vi "DDS_updateManualSettings.vi"() -> ()   [LabVIEW 2012, in "DDS9954_v2013.lvlib"]
uses:
  DDS9954_v2013.lvlib
panel:
  out "FT_Status":u32[](array[numeric])
  out "Bytes Written":u32[](array[numeric])
  in  "Program All DDS?":bool
  in  "Manual Settings Array":T1(array[cluster])=[{"Manual Frequency (MHz)"=110.0, "Manual Amplitude (0-1)"=0.38, "Max Locked Amplitude (0-1)"=0.38, "PD Set-Point (V)"=1.1, "Photodiode Offset (V)"=0.0, "P Gain (-2^8 to 2^8)"=0, "I Gain (-2^8 to 2^8)"=255, "Device Description"="Ultracool FPGA 04", "Gain Divisor (shift << by xBits))"=10, "Nickname"="Dipole 1"}, {"Manual Frequency (MHz)"=75.2, "Manual Amplitude (0-1)"=0.55, "Max Locked Amplitude (0-1)"=0.55, "PD Set-Point (V)"=1.2, "Photodiode Offset (V)"=0.0, "P Gain (-2^8 to 2^8)"=0, "I Gain (-2^8 to 2^8)"=255, "Device Description"="Ultracool FPGA 08", "Gain Divisor (shift << by xBits))"=10, "Nickname"="Dipole 2"}, {"Manual Frequency (MHz)"=92.97, "Manual Amplitude (0-1)"=0.34, "Max Locked Amplitude (0-1)"=0.34, "PD Set-Point (V)"=2.06, "Photodiode Offset (V)"=0.0, "P Gain (-2^8 to 2^8)"=0, "I Gain (-2^8 to 2^8)"=250, "Device Description"="Ultracool FPGA 05", "Gain Divisor (shift << by xBits))"=10, "Nickname"="x-y lattice"}, {"Manual Frequency (MHz)"=91.7, "Manual Amplitude (0-1)"=0.25, "Max Locked Amplitude (0-1)"=0.25, "PD Set-Point (V)"=0.46, "Photodiode Offset (V)"=0.0, "P Gain (-2^8 to 2^8)"=0, "I Gain (-2^8 to 2^8)"=250, "Device Description"="Ultracool FPGA 06", "Gain Divisor (shift << by xBits))"=10, "Nickname"="vertical lattice"}, {"Manual Frequency (MHz)"=0.0, "Manual Amplitude (0-1)"=0.0, "Max Locked Amplitude (0-1)"=0.0, "PD Set-Point (V)"=0.0, "Photodiode Offset (V)"=0.0, "P Gain (-2^8 to 2^8)"=0, "I Gain (-2^8 to 2^8)"=0, "Device Description"="Ultracool FPGA 03", "Gain Divisor (shift << by xBits))"=10, "Nickname"="RF"}, {"Manual Frequency (MHz)"=0.0, "Manual Amplitude (0-1)"=0.0, "Max Locked Amplitude (0-1)"=0.0, "PD Set-Point (V)"=0.0, "Photodiode Offset (V)"=0.0, "P Gain (-2^8 to 2^8)"=0, "I Gain (-2^8 to 2^8)"=0, "Device Description"="Ultracool FPGA 07", "Gain Divisor (shift << by xBits))"=10, "Nickname"="uW Primary"}, {"Manual Frequency (MHz)"=110.0, "Manual Amplitude (0-1)"=0.38, "Max Locked Amplitude (0-1)"=0.38, "PD Set-Point (V)"=1.1, "Photodiode Offset (V)"=0.0, "P Gain (-2^8 to 2^8)"=0, "I Gain (-2^8 to 2^8)"=255, "Device Description"="FPGA 13 uW2", "Gain Divisor (shift << by xBits))"=10, "Nickname"="uW Aux"}, {"Manual Frequency (MHz)"=80.0, "Manual Amplitude (0-1)"=0.0, "Max Locked Amplitude (0-1)"=0.0, "PD Set-Point (V)"=0.0, "Photodiode Offset (V)"=0.0, "P Gain (-2^8 to 2^8)"=0, "I Gain (-2^8 to 2^8)"=0, "Device Description"="Ultracool FPGA", "Gain Divisor (shift << by xBits))"=10, "Nickname"="Running Lattice 1"}, {"Manual Frequency (MHz)"=120.0, "Manual Amplitude (0-1)"=0.33, "Max Locked Amplitude (0-1)"=0.33, "PD Set-Point (V)"=0.0, "Photodiode Offset (V)"=0.0, "P Gain (-2^8 to 2^8)"=0, "I Gain (-2^8 to 2^8)"=0, "Device Description"="FPGA 10 780 Lattice 2", "Gain Divisor (shift << by xBits))"=10, "Nickname"="Running Lattice 2"}, {"Manual Frequency (MHz)"=0.0, "Manual Amplitude (0-1)"=0.0, "Max Locked Amplitude (0-1)"=0.0, "PD Set-Point (V)"=0.0, "Photodiode Offset (V)"=0.0, "P Gain (-2^8 to 2^8)"=0, "I Gain (-2^8 to 2^8)"=0, "Device Description"="FPGA 09", "Gain Divisor (shift << by xBits))"=10, "Nickname"="Bonus FPGA 1"}] {"Manual Frequency (MHz)" min=0.0 max=200.0; "Manual Amplitude (0-1)" min=0.0 max=1.0; "Max Locked Amplitude (0-1)" min=0.0 max=1.0; "PD Set-Point (V)" min=0.0 max=3.3; "Photodiode Offset (V)" min=0.0 max=3.3; "P Gain (-2^8 to 2^8)" min=0 max=255 step=1; "I Gain (-2^8 to 2^8)" min=0 max=255 step=1; "Gain Divisor (shift << by xBits))" max=10 step=1}
  in  "Use DDS display equivalent?":bool
  out "error out":errorcluster
  out "Characters to FPGA":string="L;004\r\nL102200242\r\nL2000034\r\nL01\r\nL411<71<720::::::;0::::::;071<71<7\r\nL615555555155555550>38>38>0>38>38>\r\nL31000100010001000\r\nL50000000000000000\r\nL70200000001010000000102000000010200000001\r\nL80200000001010000000102000000010200000001\r\nL:0;>;<2000;>;<2000;>;<2000;>;<200\r\nL91010\r\n"
  # "Program will reprogram first displayed FPGA device in the array\nAlternatively, program can reprogram ALL FPGA devices by clicking the option"
  # "Nicknames:\nUltracool FPGA 03 = RF\nUltracool FPGA 04 = Dipole 1\nUltracool FPGA 07 = uW 1\nUltracool FPGA 08 = Dipole 2\nFPGA 13 uW2 = uW 2"
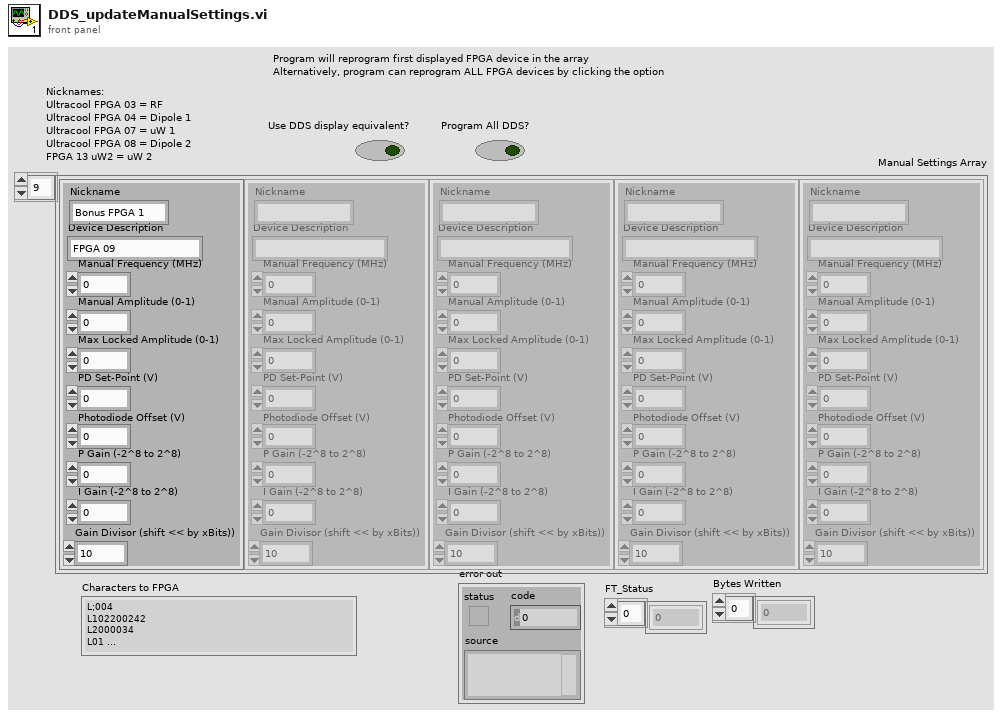
[diagram p1: front panel]
types:
  T1 = cluster{"Manual Frequency (MHz)":dbl, "Manual Amplitude (0-1)":dbl, "Max Locked Amplitude (0-1)":dbl, "PD Set-Point (V)":dbl, "Photodiode Offset (V)":dbl, "P Gain (-2^8 to 2^8)":i16, "I Gain (-2^8 to 2^8)":i16, "Device Description":string, "Gain Divisor (shift << by xBits))":u8, "Nickname":string}[]
  T2 = cluster{"Manual Frequency (MHz)":dbl, "Manual Amplitude (0-1)":dbl, "Max Locked Amplitude (0-1)":dbl, "PD Set-Point (V)":dbl, "Photodiode Offset (V)":dbl, "P Gain (-2^8 to 2^8)":i16, "I Gain (-2^8 to 2^8)":i16, "Device Description":string, "Gain Divisor (shift << by xBits))":u8, "Nickname":string}
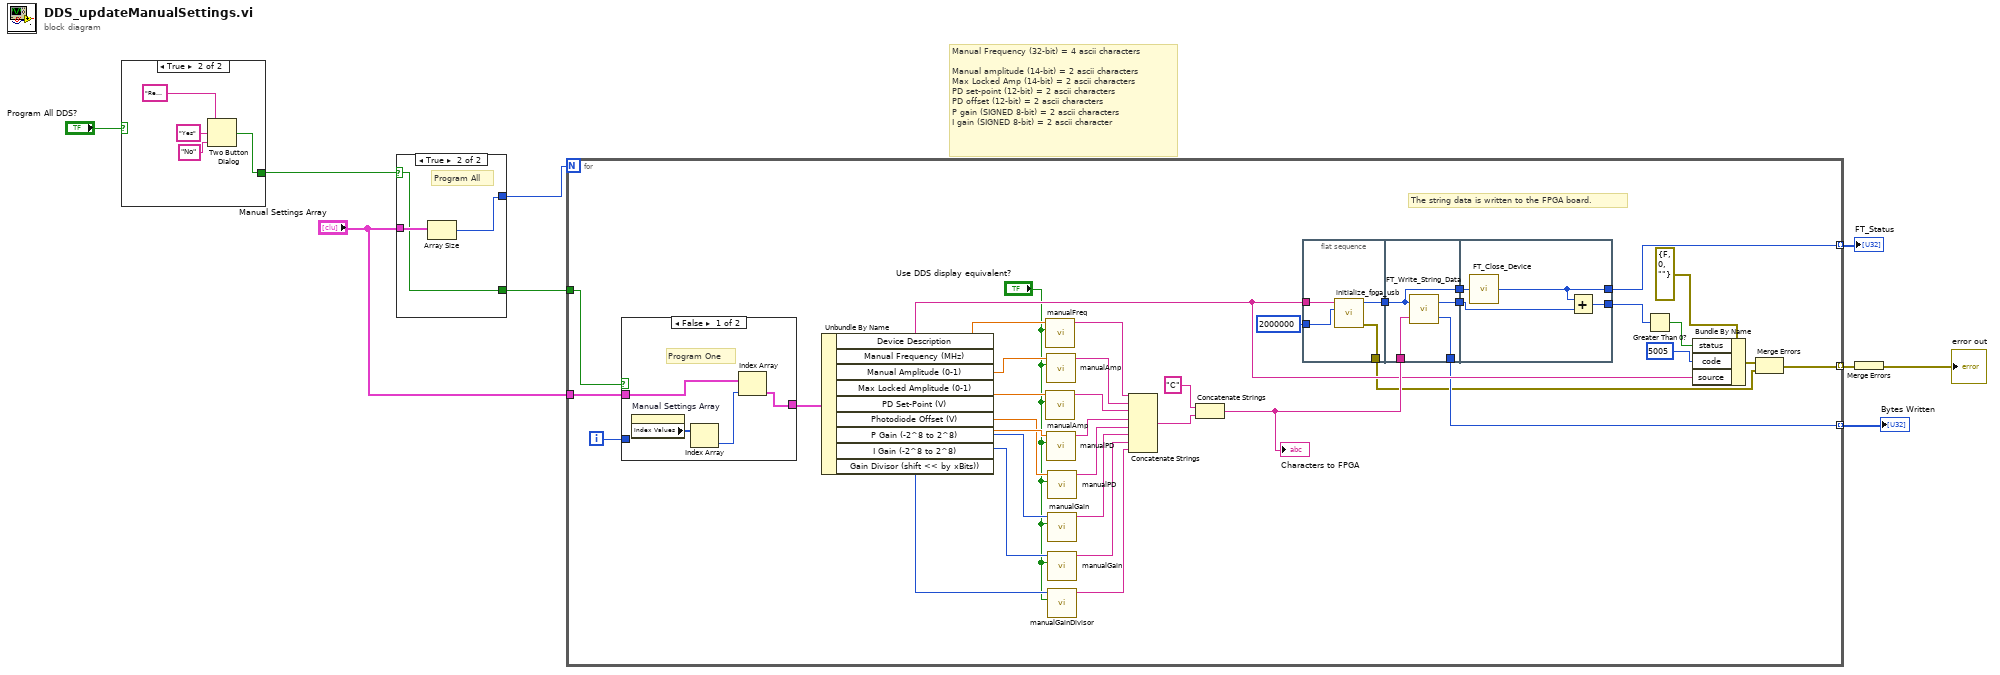
[diagram p0: block diagram]
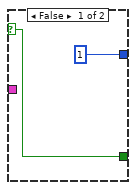
[diagram p3: hidden frame]
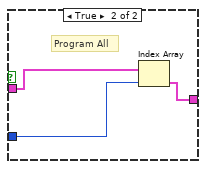
[diagram p4: hidden frame]
diagram:
  # "Manual Frequency (32-bit) = 4 ascii characters\n\nManual amplitude (14-bit) = 2 ascii characters\nMax Locked Amp (14-bit) = 2 ascii characters\nPD set-point (12-bit) = 2 ascii characters\nPD offset (12-bit) = 2 ascii characters\nP gain (SIGNED 8-bit) = 2 ascii characters\nI gain (SIGNED 8-bit) = 2 ascii character"
  n1 = case shown="True" "Program All DDS?" {
    selector: "Program All DDS?" -> [w10 _]
    tunnel: [w10 w14] -> w5
    frame False {
    }
    frame True {
      n2 = Two Button Dialog(message="Really reprogram ALL FPGAs in the array?", 1:"No" ("F button name (\"Cancel\")"), 2:"Yes" ("T button name (\"OK\")")) -> (T button?=w14:bool)
    }
  }
  n3 = case shown="True" w5 {
    selector: w5 -> [w15 w17]
    tunnel: "Manual Settings Array" -> [_ w19]
    tunnel: [1 w18] -> w9
    tunnel: [w15 w17] -> w8
    frame False {
    }
    frame True {
      # "Program All"
      n4 = Array Size(array=w19) -> (size(s)=w18:i32)
    }
  }
  n5 = for {
    N: w9 -> [_]
    tunnel: [w50] -> w4 mode=indexing
    tunnel: [w45] -> w2 mode=indexing
    tunnel: [w25] -> w3 mode=indexing
    tunnel: w8 -> [w23]
    tunnel: "Manual Settings Array" -> [w22]
    i -> [w20]
    # "The string data is written to the FPGA board."
    n6 = case shown="False" w23 {
      tunnel: w22 -> [w60 w64]
      tunnel: [w59 w62] -> w21
      tunnel: w20 -> [_ w63]
      frame False {
        # "Program One"
        n7 = property on="Manual Settings Array" class="Arr (strict)"() -> ("Index Values"=w61:u32[])  [unwired: 2 in, 2 out]
        n8 = Index Array(array=w61) -> (element=w58:u32)  [unwired: 1 in]
        n9 = Index Array(array=w60, index=w58) -> (element=w59:T2)
      }
      frame True {
        # "Program All"
        n10 = Index Array(array=w64, index=w63) -> (element=w62:T2)
      }
    }
    n11 = Unbundle By Name(w21) -> ("Device Description"=w51:string, "Manual Frequency (MHz)"=w41:dbl, "Manual Amplitude (0-1)"=w39:dbl, "Max Locked Amplitude (0-1)"=w38:dbl, "PD Set-Point (V)"=w36:dbl, "Photodiode Offset (V)"=w34:dbl, "P Gain (-2^8 to 2^8)"=w31:i16, "I Gain (-2^8 to 2^8)"=w29:i16, "Gain Divisor (shift << by xBits))"=w32:u8)
    n12 = call "manualFreq.vi"("Use DDS display equivalent?"="Use DDS display equivalent?", "Manual Frequency (MHz)"=w41) -> ("Frequency string out"=w40:string)  [unwired: 8 in, 1 out]
    n13 = call "manualAmp.vi"("Use DDS display equivalent?"="Use DDS display equivalent?", "Manual Amplitude (0-1)"=w38) -> ("Amplitude string out"=w37:string)  [unwired: 8 in, 1 out]
    n14 = call "manualAmp.vi"("Use DDS display equivalent?"="Use DDS display equivalent?", "Manual Amplitude (0-1)"=w39) -> ("Amplitude string out"=w26:string)  [unwired: 8 in, 1 out]
    n15 = call "manualPD.vi"("Use DDS display equivalent?"="Use DDS display equivalent?", "Manual Photodiode (V)"=w36) -> ("Photodiode string out"=w35:string)  [unwired: 8 in, 1 out]
    n16 = call "manualPD.vi"("Use DDS display equivalent?"="Use DDS display equivalent?", "Manual Photodiode (V)"=w34) -> ("Photodiode string out"=w33:string)  [unwired: 8 in, 1 out]
    n17 = call "manualGain.vi"("Use DDS display equivalent?"="Use DDS display equivalent?", "Gain (arb)"=w31) -> ("Photodiode string out"=w30:string)  [unwired: 8 in, 1 out]
    n18 = call "manualGain.vi"("Use DDS display equivalent?"="Use DDS display equivalent?", "Gain (arb)"=w29) -> ("Photodiode string out"=w28:string)  [unwired: 8 in, 1 out]
    n19 = call "manualGainDivisor.vi"("Use DDS display equivalent?"="Use DDS display equivalent?", "Gain Divisor (number of bits to shift)"=w32) -> ("Gain divisor string out"=w24:string)  [unwired: 8 in, 1 out]
    n20 = Concatenate Strings(w40, w26, w37, w35, w33, w30, w28, w24) -> (w53:string)
    n21 = Concatenate Strings("C" ("string"), w53) -> (w52:string)
    "Characters to FPGA" <- w52
    n22 = flat-sequence {
      tunnel: [w68] -> w57
      tunnel: w51 -> [w67]
      tunnel: u32 2000000 ("Baud Rate") -> [w66]
      tunnel: [w65] -> w44
      tunnel: w57 -> [w69]
      tunnel: [w72] -> w50
      tunnel: w52 -> [w71]
      tunnel: [w69] -> w56
      tunnel: [w70] -> w55
      tunnel: w56 -> [w76]
      tunnel: [w75] -> w25
      tunnel: w55 -> [w74]
      tunnel: [w73] -> w46
      frame #0 {
        n23 = call "initialize_fpga_usb.vi"("Baud Rate"=w66, "Device Description"=w67) -> ("error out"=w65:errorcluster, "Handle"=w68:u32)  [unwired: 4 in]
      }
      frame #1 {
        n24 = call "FT_Write_String_Data.vi"("Buffer"=w71, "Handle"=w69) -> ("Bytes Written"=w72:u32, "FT_Status"=w70:u32)
      }
      frame #2 {
        n25 = call "FT_Close_Device.vi"("Handle"=w76) -> ("FT_Status"=w75:u32)
        n26 = Add(x=w75, y=w74) -> (x+y=w73:u32)
      }
    }
    n27 = Greater Than 0?(x=w46) -> (x > 0?=w47:bool)
    n28 = Bundle By Name(cluster=errorcluster {"status"=FALSE, "code"=0, "source"=""} ("error constant"), "status"=w47, "code"=5005, "source"=w51) -> (w43:errorcluster)
    n29 = Merge Errors(w43, w44) -> (w45:errorcluster)
  }
  "Bytes Written" <- w4
  "FT_Status" <- w3
  n30 = Merge Errors(w2) -> (→"error out":errorcluster)
